vi "SimulatedSignalConfig.vi"() -> ()   [LabVIEW 2017, in "EmsaAcquisition.lvlib"]
uses:
  <vilib>/addons/InsightCM/Devices/Shared/Emsa/EmsaAcquisition/EmsaAcquisition.lvlib
  <vilib>/addons/InsightCM/Devices/Shared/Emsa/EmsaAcquisition/controls/SimulatedSignalConfig.ctl
  <vilib>/addons/InsightCM/Devices/Shared/Emsa/EmsaAcquisition/controls/SimulatedSweepConfig.ctl
  <vilib>/addons/InsightCM/Devices/Shared/Emsa/EmsaAcquisition/controls/SweepElement.ctl
  <vilib>/addons/InsightCM/Devices/Shared/Emsa/EmsaAcquisition/controls/SimulatedConfigRefs.ctl
  <vilib>/addons/InsightCM/Devices/Shared/Emsa/EmsaAcquisition/subVIs/SimulatedConfigRefGlobal.vi
panel:
  in  "SimulatedSignalConfig":T1
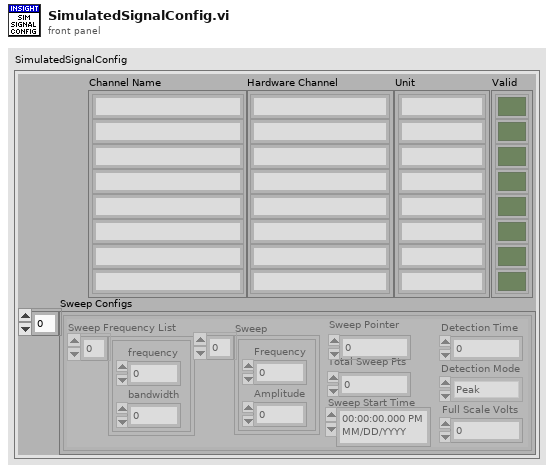
[diagram p1: front panel]
types:
  T1 = typedef "EmsaAcquisition.lvlib/SimulatedSignalConfig.ctl" = cluster{"Channel Name":string[], "Valid":bool[], "Hardware Channel":string[], "Unit":string[], "Sweep Configs":T2[]}
  T2 = typedef "EmsaAcquisition.lvlib/SimulatedSweepConfig.ctl" = cluster{"Sweep Frequency List":cluster{"frequency":dbl, "bandwidth":dbl}[], "Detection Time":dbl, "Detection Mode":enum16{"Peak", "Quasi Peak", "Average"}, "Full Scale Volts":dbl, "Total Sweep Pts":i32, "Sweep Pointer":i32, "Sweep":T3[], "Sweep Start Time":timestamp}
  T3 = typedef "EmsaAcquisition.lvlib/SweepElement.ctl" = cluster{"Frequency":dbl, "Amplitude":dbl}
  T4 = typedef "EmsaAcquisition.lvlib/SimulatedConfigRefs.ctl" = cluster{"SimulatedSignalConfig":refnum<vi>}
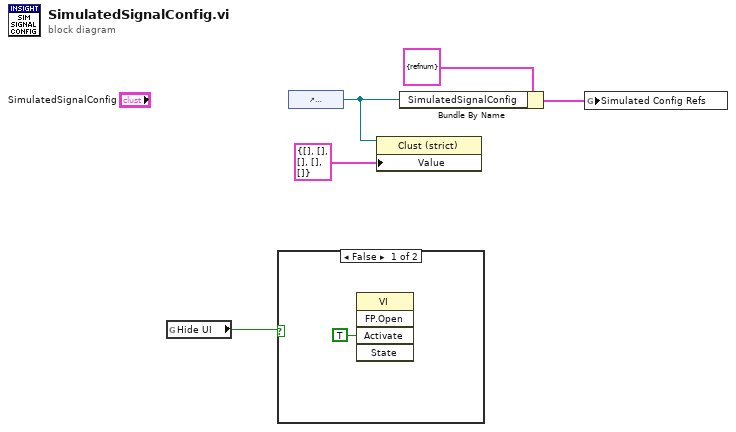
[diagram p0: block diagram]
diagram:
  n1 = global read "SimulatedConfigRefGlobal.vi" "Hide UI"() -> (w5:bool)
  n2 = case shown="False" w5 {
    frame False {
      n3 = invoke class="VI" method="FP.Open"("Activate"=TRUE ("Activate?")) -> ()  [unwired: 4 in, 5 out]
    }
    frame True {
    }
  }
  n4 = control-ref of="SimulatedSignalConfig"() -> (w1:refnum<vi>)
  n5 = property class="Clust (strict)"(reference=w1, "Value"=T1 {"Channel Name"=[], "Valid"=[], "Hardware Channel"=[], "Unit"=[], "Sweep Configs"=[]}) -> ()  [unwired: 1 in, 2 out]
  n6 = Bundle By Name(cluster=T4 {"SimulatedSignalConfig"=refnum} ("Simulated Config Refs"), "SimulatedSignalConfig"=w1) -> (w4:T4)
  n7 = global write "SimulatedConfigRefGlobal.vi" "Simulated Config Refs"(w4) -> ()
